vi "Signal(Int16)ToNode(viaString).vi"(0 "Tree DVR in":refnum<data-value>, 1 "NodePath":string, 2 "y-axis (Data Range)":i16[](array[numeric]), 3 "Start Time":dbl, 4 "Delta t":dbl, 5 "Error in":errorcluster) -> (6 "Tree DVR out":refnum<data-value>, 8 "Error out":errorcluster)   [LabVIEW 2014]
uses:
  <vilib>/MDSplus/Classes/Tree_Class/Tree.lvclass
  <vilib>/MDSplus/Library/MDSplus.lvlib
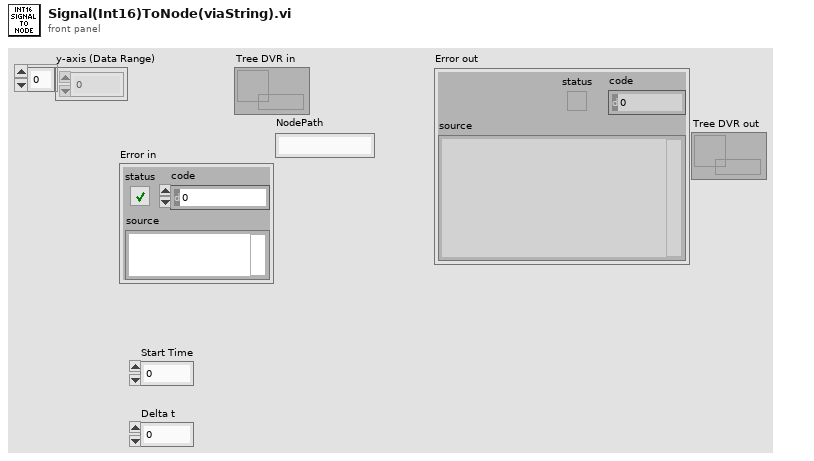
[diagram p1: front panel]
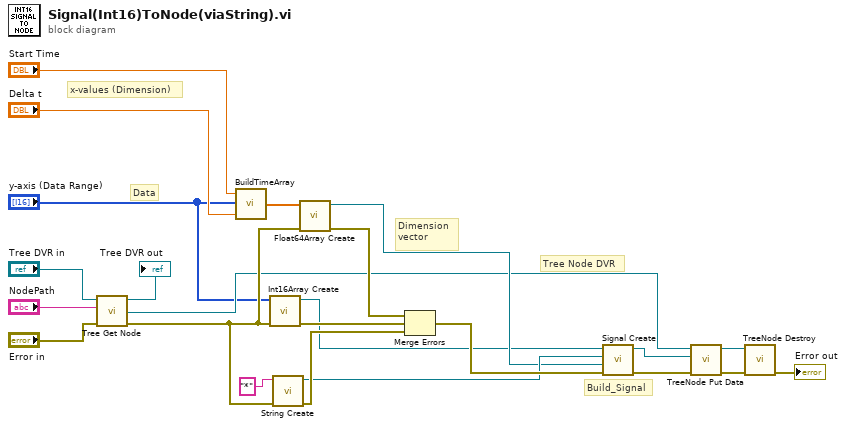
[diagram p0: block diagram]
diagram:
  # "Build_Signal"
  # "Dimension vector"
  # "x-values (Dimension)"
  # "Tree Node DVR"
  # "Data"
  n1 = call <vilib>:"Tree Get Node.vi"("error in (no error)"="Error in", "Path"="NodePath", "Tree DVR in"="Tree DVR in") -> ("error out"=w10:errorcluster, "Node out"=w5:refnum<data-value>, "Tree DVR out"=→"Tree DVR out":refnum<data-value>)  [unwired: 6 in]
  n2 = call "BuildTimeArray.vi"("Time Increment (dt)"="Delta t", "Data Array (y-values)"="y-axis (Data Range)", "Start Time (t_o)"="Start Time") -> ("Time Array (x-values)"=w14:dbl[])
  n3 = call <vilib>:"Int16Array Create.vi"("error in (no error)"=w10, "I16 array in"="y-axis (Data Range)") -> ("error out"=w18:errorcluster, "Int16Array DVR out"=w7:refnum<data-value>)  [unwired: 8 in]
  n4 = call <vilib>:"String Create.vi"("error in (no error)"=w10, "String value in"="*") -> ("error out"=w11:errorcluster, "String DVR out"=w9:refnum<data-value>)  [unwired: 8 in]
  n5 = call <vilib>:"Float64Array Create.vi"("error in (no error)"=w10, "DBL array in"=w14) -> ("error out"=w13:errorcluster, "Float64Array DVR out"=w8:refnum<data-value>)  [unwired: 8 in]
  n6 = Merge Errors(w13, w18, w11) -> (w17:errorcluster)
  n7 = call <vilib>:"Signal Create.vi"("error in (no error)"=w17, "Dimension"=w8, "Raw"=w9, "Data"=w7) -> ("error out"=w19:errorcluster, "Signal DVR out"=w6:refnum<data-value>)  [unwired: 6 in]
  n8 = call <vilib>:"TreeNode Put Data.vi"("error in (no error)"=w19, "Data"=w6, "TreeNode DVR in"=w5) -> ("error out"=w2:errorcluster, "TreeNode DVR out"=w3:refnum<data-value>)  [unwired: 7 in]
  n9 = call <vilib>:"TreeNode Destroy.vi"("error in (no error)"=w2, "TreeNode DVR in"=w3) -> ("error out"=→"Error out":errorcluster)  [unwired: 9 in]
